vi "putFtp.vi"(8 "host":string="10.8.62.12", 10 "local path":path=path "C:/_CODE/ini/test.ini", 11 "remote path":string="/home/lvuser/calibrations/test2.ini") -> (0 "file error out":errorcluster, 3 "ftp error out 2":errorcluster)   [LabVIEW 2014]
uses:
  <vilib>/FTP/NI_FTP.lvlib
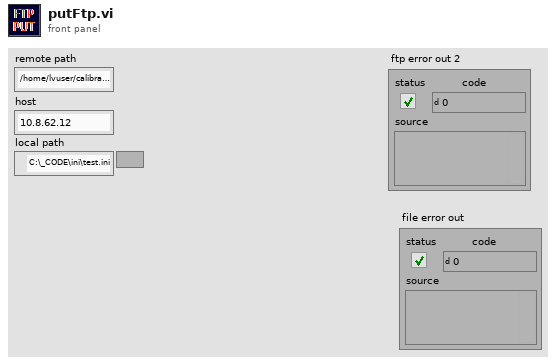
[diagram p1: front panel]
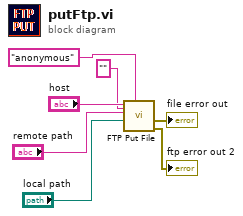
[diagram p0: block diagram]
diagram:
  n1 = call <vilib>:"FTP Put File.vi"("password"="", "user"="anonymous", "local path"="local path", "remote path"="remote path", "host"="host") -> ("error out"=→"ftp error out 2":errorcluster, "file error"=→"file error out":errorcluster)  [unwired: 5 in]
